vi "Get Column From Index.vi"(1 "array":string[][](array[string]), 2 "index":i32) -> (0 "subarray":string[](array[string]))   [LabVIEW 2018]
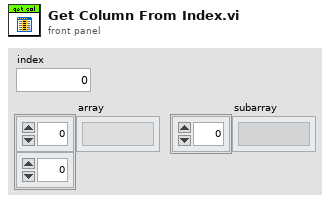
[diagram p1: front panel]
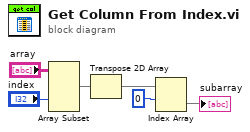
[diagram p0: block diagram]
diagram:
  n1 = Array Subset(array="array", index (col)="index") -> (w6:string[][])  [unwired: 3 in]
  n2 = Transpose 2D Array(2D array=w6) -> (transposed array=w5:string[][])
  n3 = Index Array(array=w5, index (row)=0) -> (element=→"subarray":string[])  [unwired: 1 in]
